vi "Mathematical operations.vi"() -> ()   [LabVIEW 2019]
panel:
  out "sqrt(x)":dbl
  out "nearest integer value":dbl
  out "x*2^n":dbl
  out "x-1":dbl
  out "x+1":dbl
  in  "Input 3":dbl
  out "floor(x/y)":dbl
  out "x-y*floor(x/y)":dbl
  out "x/y":dbl
  out "x*y":dbl
  out "x-y":dbl
  in  "Input\n 2":dbl
  in  "Input 1":dbl
  out "x+y":dbl
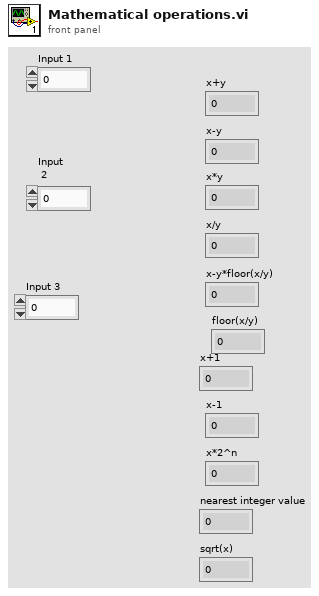
[diagram p1: front panel]
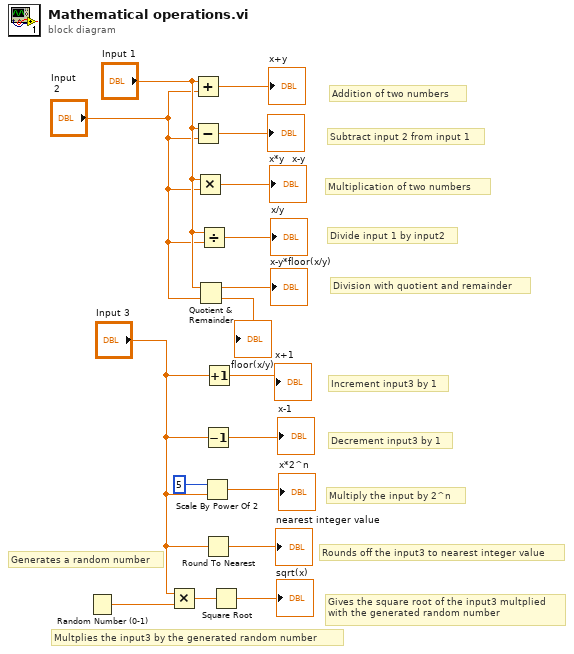
[diagram p0: block diagram]
diagram:
  # "Multplies the input3 by the generated random number"
  # "Generates a random number"
  # "Gives the square root of the input3 multplied\nwith the generated random number"
  # "Rounds off the input3 to nearest integer value"
  # "Multiply the input by 2^n"
  # "Decrement input3 by 1"
  # "Increment input3 by 1"
  # "Division with quotient and remainder"
  # "Divide input 1 by input2"
  # "Multiplication of two numbers"
  # "Subtract input 2 from input 1"
  # "Addition of two numbers"
  n1 = Random Number (0-1)() -> (number: 0 to 1=w3:dbl)
  n2 = Multiply(x="Input 3", y=w3) -> (x*y=w2:dbl)
  n3 = Add(x="Input 1", y="Input\n 2") -> (x+y=→"x+y":dbl)
  n4 = Subtract(x="Input 1", y="Input\n 2") -> (x-y=→"x-y":dbl)
  n5 = Multiply(x="Input 1", y="Input\n 2") -> (x*y=→"x*y":dbl)
  n6 = Quotient & Remainder(x="Input 1", y="Input\n 2") -> (x-y*floor(x/y)=→"x-y*floor(x/y)":dbl, floor(x/y)=→"floor(x/y)":dbl)
  n7 = Divide(x="Input 1", y="Input\n 2") -> (x/y=→"x/y":dbl)
  n8 = Scale By Power Of 2(n=5, x="Input 3") -> (x*2^n=→"x*2^n":dbl)
  n9 = Decrement(x="Input 3") -> (x-1=→"x-1":dbl)
  n10 = Round To Nearest(number="Input 3") -> (nearest integer value=→"nearest integer value":dbl)
  n11 = Increment(x="Input 3") -> (x+1=→"x+1":dbl)
  n12 = Square Root(x=w2) -> (sqrt(x)=→"sqrt(x)":dbl)
